vi "Abort Auto Test Global.vi"() -> ()   [LabVIEW 2015]
panel:
  in  "Abort Auto Test":bool
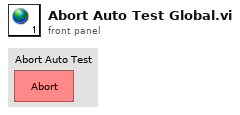
[diagram p1: front panel]
diagram:
